vi "关键参数转data(子VI).vi"(10 "改变?":bool, 11 "关键参数":T1) -> (3 "数组":string[][](array[string]))   [LabVIEW 2016, in "数据传输系统-02.lvlib"]
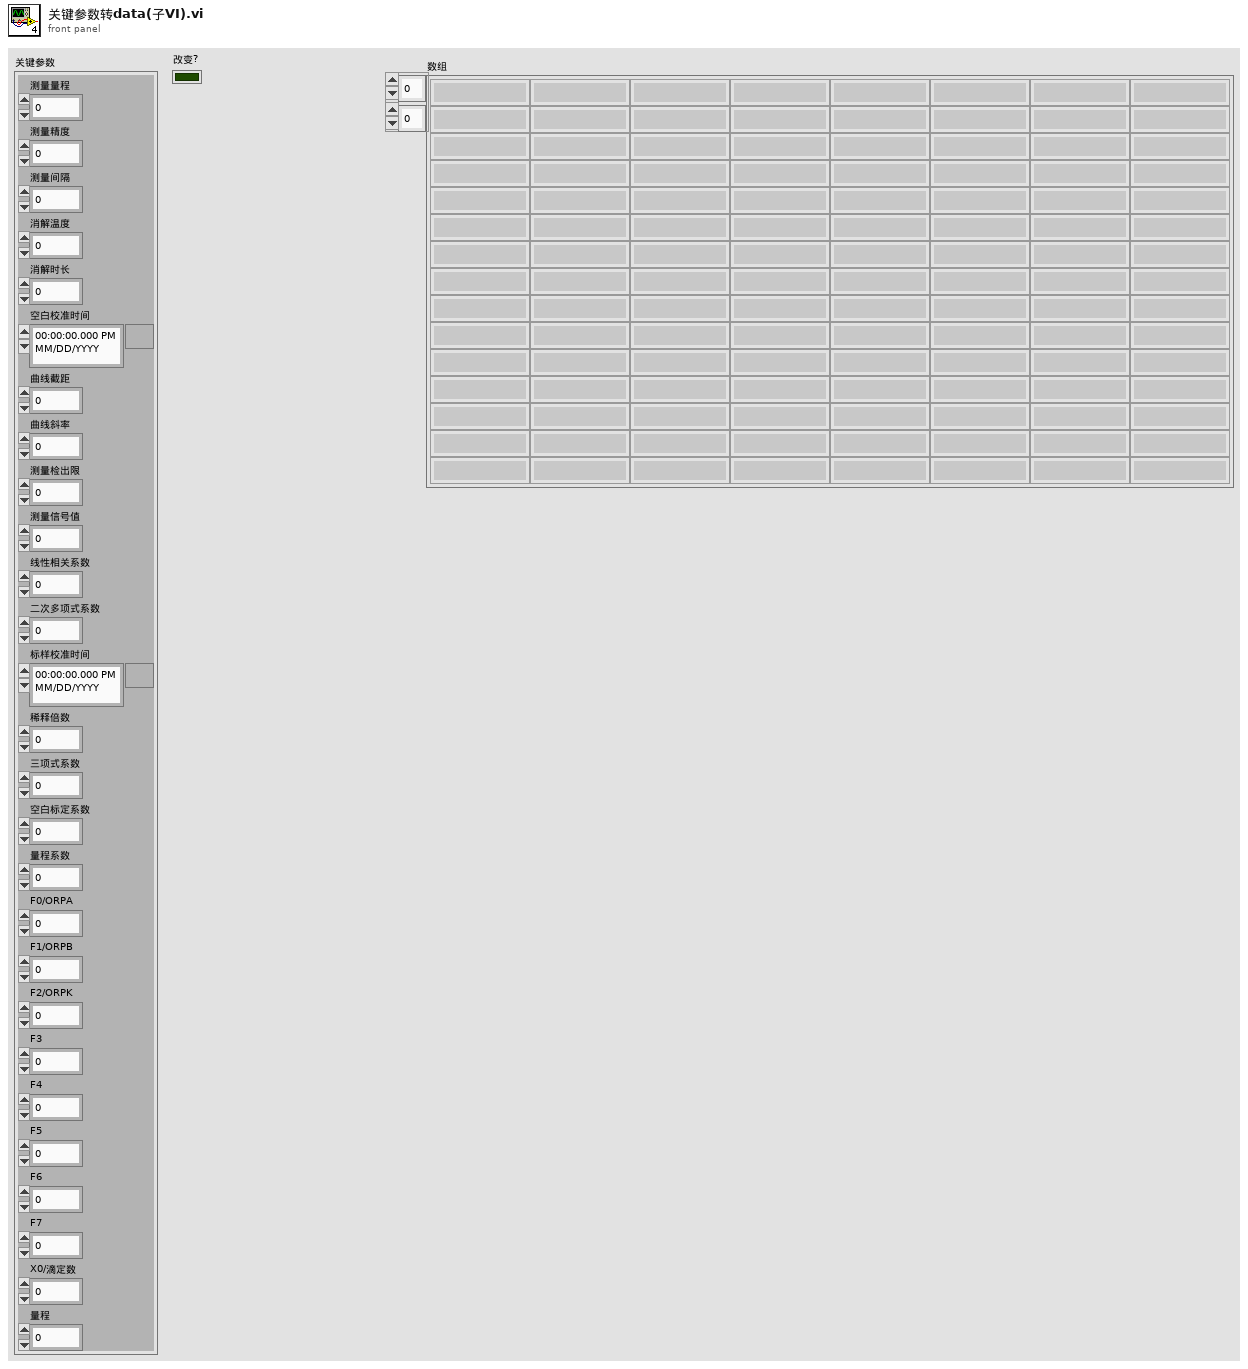
[diagram p1: front panel]
types:
  T1 = cluster{"测量量程":dbl, "测量精度":dbl, "测量间隔":dbl, "消解温度":dbl, "消解时长":dbl, "空白校准时间":timestamp, "曲线截距":dbl, "曲线斜率":dbl, "测量检出限":dbl, "测量信号值":dbl, "线性相关系数":dbl, "二次多项式系数":dbl, "标样校准时间":timestamp, "稀释倍数":dbl, "三项式系数":dbl, "空白标定系数":dbl, "量程系数":dbl, "F0/ORPA":dbl, "F1/ORPB":dbl, "F2/ORPK":dbl, "F3":dbl, "F4":dbl, "F5":dbl, "F6":dbl, "F7":dbl, "X0/滴定数":dbl, "量程":dbl}
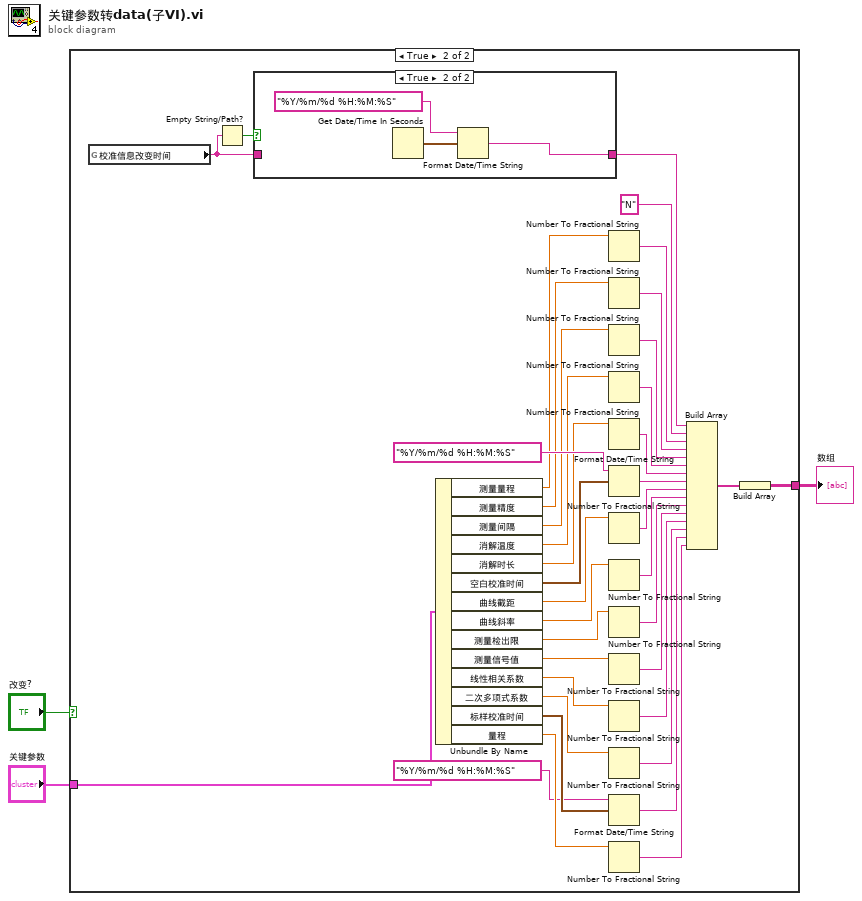
[diagram p0: block diagram]
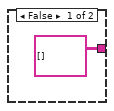
[diagram p2: hidden frame]
diagram:
  n1 = case shown="True" "改变?" {
    tunnel: [string[][] [] w41] -> w3
    tunnel: "关键参数" -> [_ w7]
    frame False {
    }
    frame True {
      n2 = global read "全局1.vi" "校准信息改变时间"() -> (w5:string)
      n3 = Empty String/Path?(string/path=w5) -> (empty?=w6:bool)
      n4 = case shown="True" w6 {
        tunnel: [w42 w45] -> w9
        tunnel: w5 -> [w42 _]
        frame False {
        }
        frame True {
          n5 = Get Date/Time In Seconds() -> (seconds since 1Jan1904=w44:timestamp)
          n6 = Format Date/Time String(time format string (%c)="%Y/%m/%d %H:%M:%S" ("时间格式字符串(%c)"), seconds (now)=w44) -> (date/time string=w45:string)  [unwired: 1 in]
        }
      }
      n7 = Unbundle By Name(w7) -> ("测量量程"=w8:dbl, "测量精度"=w12:dbl, "测量间隔"=w14:dbl, "消解温度"=w16:dbl, "消解时长"=w18:dbl, "空白校准时间"=w21:timestamp, "曲线截距"=w23:dbl, "曲线斜率"=w24:dbl, "测量检出限"=w25:dbl, "测量信号值"=w26:dbl, "线性相关系数"=w27:dbl, "二次多项式系数"=w28:dbl, "标样校准时间"=w30:timestamp, "量程"=w31:dbl)
      n8 = Number To Fractional String(number=w8) -> (F-format string=w11:string)  [unwired: 3 in]
      n9 = Number To Fractional String(number=w12) -> (F-format string=w13:string)  [unwired: 3 in]
      n10 = Number To Fractional String(number=w14) -> (F-format string=w15:string)  [unwired: 3 in]
      n11 = Number To Fractional String(number=w16) -> (F-format string=w17:string)  [unwired: 3 in]
      n12 = Number To Fractional String(number=w18) -> (F-format string=w19:string)  [unwired: 3 in]
      n13 = Format Date/Time String(time format string (%c)="%Y/%m/%d %H:%M:%S" ("时间格式字符串(%c)"), seconds (now)=w21) -> (date/time string=w22:string)  [unwired: 1 in]
      n14 = Number To Fractional String(number=w23) -> (F-format string=w32:string)  [unwired: 3 in]
      n15 = Number To Fractional String(number=w24) -> (F-format string=w33:string)  [unwired: 3 in]
      n16 = Number To Fractional String(number=w25) -> (F-format string=w34:string)  [unwired: 3 in]
      n17 = Number To Fractional String(number=w26) -> (F-format string=w35:string)  [unwired: 3 in]
      n18 = Number To Fractional String(number=w27) -> (F-format string=w36:string)  [unwired: 3 in]
      n19 = Number To Fractional String(number=w28) -> (F-format string=w37:string)  [unwired: 3 in]
      n20 = Format Date/Time String(time format string (%c)="%Y/%m/%d %H:%M:%S" ("时间格式字符串(%c)"), seconds (now)=w30) -> (date/time string=w38:string)  [unwired: 1 in]
      n21 = Number To Fractional String(number=w31) -> (F-format string=w39:string)  [unwired: 3 in]
      n22 = Build Array(w9, "N", w11, w13, w15, w17, w19, w22, w32, w33, w34, w35, w36, w37, w38, w39) -> (w40:string[])
      n23 = Build Array(w40) -> (w41:string[][])
    }
  }
  "数组" <- w3
